vi "PH_AWG-510.read Output Settings from String Data File.vi"(1 "Data File String":string) -> (0 "Output Settings":T1={"Activate Channel"=FALSE, "VPP (V)"=0.0, "Clock (Hz)"=0.0, "File Name (Device)"="", "#1"=0, "#2"=0, "#3"=0, "#4"=0, "#5"=0, "#6"=0, "#7"=0, "#8"=0, "#9"=0, "#10"=0, "#11"=0, "#12"=0, "#13"=0, "#14"=0, "#15"=0, "#16"=0, "#17"=0, "#18"=0, "#19"=0, "#20"=0, "Offset (V)"=-1.0} {"#20" max=1023 step=1 scale=0.0..1023.0; "#19" max=1023 step=1 scale=0.0..1023.0; "#18" max=1023 step=1 scale=0.0..1023.0; "#17" max=1023 step=1 scale=0.0..1023.0; "#16" max=1023 step=1 scale=0.0..1023.0; "#15" max=1023 step=1 scale=0.0..1023.0; "#14" max=1023 step=1 scale=0.0..1023.0; "#13" max=1023 step=1 scale=0.0..1023.0; "#12" max=1023 step=1 scale=0.0..1023.0; "#11" max=1023 step=1 scale=0.0..1023.0; "#10" max=1023 step=1 scale=0.0..1023.0; "#9" max=1023 step=1 scale=0.0..1023.0; "#8" max=1023 step=1 scale=0.0..1023.0; "#7" max=1023 step=1 scale=0.0..1023.0; "#6" max=1023 step=1 scale=0.0..1023.0; "#5" max=1023 step=1 scale=0.0..1023.0; "#4" max=1023 step=1 scale=0.0..1023.0; "#3" max=1023 step=1 scale=0.0..1023.0; "#2" max=1023 step=1 scale=0.0..1023.0; "#1" max=1023 step=1 scale=0.0..1023.0})   [LabVIEW 2014, in "PH_AWG-510.lvlib"]
uses:
  PH_AWG-510.lvlib
  PH_AWG-510.Output Settings.ctl
panel:
  # "Waveform Pattern"
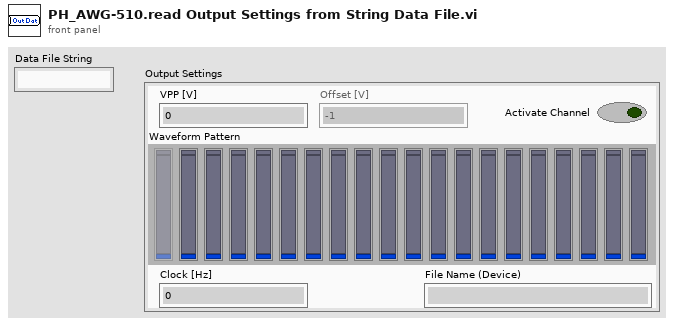
[diagram p1: front panel]
types:
  T1 = typedef "PH_AWG-510.lvlib/PH_AWG-510.Output Settings.ctl" = cluster{"Activate Channel":bool, "VPP (V)":dbl, "Clock (Hz)":dbl, "File Name (Device)":string, "#1":u16, "#2":u16, "#3":u16, "#4":u16, "#5":u16, "#6":u16, "#7":u16, "#8":u16, "#9":u16, "#10":u16, "#11":u16, "#12":u16, "#13":u16, "#14":u16, "#15":u16, "#16":u16, "#17":u16, "#18":u16, "#19":u16, "#20":u16, "Offset (V)":dbl}
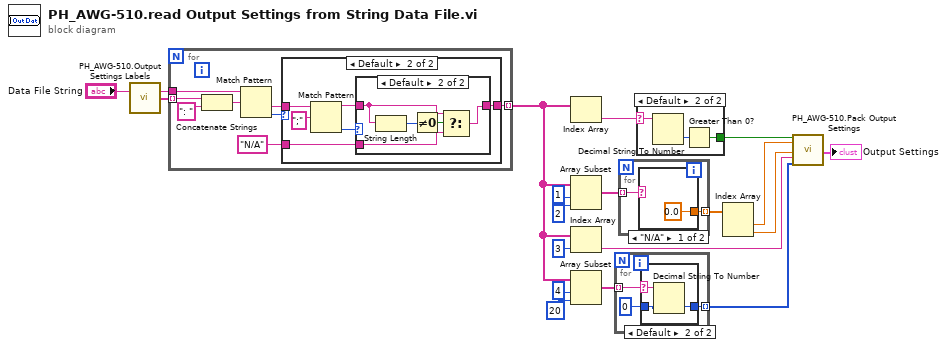
[diagram p0: block diagram]
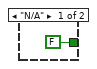
[diagram p2: hidden frame]
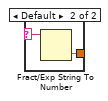
[diagram p3: hidden frame]
diagram:
  n1 = call "PH_AWG-510.Output Settings Labels.vi"() -> ("Output Settings Labels"=w18:string[])
  n2 = for {
    tunnel: "Data File String" -> [w26]
    tunnel: w18 -> [w24] mode=indexing
    tunnel: [w20] -> w6 mode=indexing
    n3 = Concatenate Strings(w24, ": " ("string")) -> (w25:string)
    n4 = Match Pattern(string=w26, regular expression=w25) -> (after substring=w21:string, offset past match=w22:i32)  [unwired: 1 in, 2 out]
    n5 = case shown="Default" w22 {
      tunnel: w21 -> [_ w33]
      tunnel: [w27 w30] -> w20
      tunnel: "N/A" -> [w27 w28]
      frame -1 {
      }
      frame Default {
        n6 = Match Pattern(string=w33, regular expression=";") -> (before substring=w29:string, offset past match=w31:i32)  [unwired: 1 in, 2 out]
        n7 = case shown="Default" w31 {
          tunnel: [w34 w35] -> w30
          tunnel: w29 -> [_ w37]
          tunnel: w28 -> [w34 w36]
          frame -1 {
          }
          frame Default {
            n8 = String Length(string=w37) -> (length=w39:i32)
            n9 = Not Equal To 0?(x=w39) -> (x != 0?=w38:bool)
            n10 = Select(t=w37, s=w38, f=w36) -> (s? t:f=w35:string)
          }
        }
      }
    }
  }
  n11 = Index Array(array=w6) -> (element=w2:string)  [unwired: 1 in]
  n12 = Array Subset(array=w6, index=1, length=2) -> (w9:string[])
  n13 = Index Array(array=w6, index=3) -> (element=w3:string)
  n14 = Array Subset(array=w6, index=4, length=20) -> (w13:string[])
  n15 = for {
    tunnel: w13 -> [w40] mode=indexing
    tunnel: [w41] -> w4 mode=indexing
    n16 = case shown="Default" w40 {
      selector: w40 -> [_ w44]
      tunnel: u16 0 ("default (0 I32)") -> [w43 w46]
      tunnel: [w43 w45] -> w41
      frame "N/A" {
      }
      frame Default {
        n17 = Decimal String To Number(string=w44, default (0L)=w46) -> (number=w45:u16)  [unwired: 1 in, 1 out]
      }
    }
  }
  n18 = for {
    tunnel: w9 -> [w47] mode=indexing
    tunnel: [w48] -> w8 mode=indexing
    n19 = case shown="\"N/A\"" w47 {
      selector: w47 -> [_ w50]
      tunnel: [0.0 w51] -> w48
      frame "N/A" {
      }
      frame Default {
        n20 = Fract/Exp String To Number(string=w50) -> (number=w51:dbl)  [unwired: 3 in, 1 out]
      }
    }
  }
  n21 = case shown="Default" w2 {
    selector: w2 -> [_ w53]
    tunnel: [FALSE w54] -> w12
    frame "N/A" {
    }
    frame Default {
      n22 = Decimal String To Number(string=w53) -> (number=w55:i32)  [unwired: 2 in, 1 out]
      n23 = Greater Than 0?(x=w55) -> (x > 0?=w54:bool)
    }
  }
  n24 = Index Array(array=w8) -> (element #1=w7:dbl, element #2=w1:dbl)  [unwired: 2 in]
  n25 = call "PH_AWG-510.Pack Output Settings.vi"("Activate Channel"=w12, "VPP [Volts]"=w7, "Clock [Hz]"=w1, "File Name"=w3, "Waveform Pattern [#1 ... #20]"=w4) -> ("Output Settings"=→"Output Settings":T1)  [unwired: 14 in]
